vi "AutobalanceTest.vi"() -> ()   [LabVIEW 2009]
uses:
  Test Utilities/DAQ Read Actions.ctl
panel:
  in  "Log Name":string="Log"
  in  "Labels":string[](array[string])=["X1", "X2", "Y1", "Z1", "Z2", "Z3"]
  in  "Start":bool
  out "Servo Error vs Command Voltage":cluster{dbl[], dbl[]}[](graph)=[{[-9.0, 9.0, -8.8, 8.8, -8.6, 8.6, -8.4, 8.4, -8.2, 8.2, -8.0, 8.0, -7.8, 7.8, -7.6, 7.6, -7.4, 7.4, -7.2, 7.2, -7.0, 7.0, -6.8, 6.8, -6.6, 6.6, -6.4, 6.4, -6.199999999999999, 6.199999999999999, -6.0, 6.0, -5.8, 5.8, -5.6, 5.6, -5.4, 5.4, -5.199999999999999, 5.199999999999999, -5.0, 5.0, -4.8, 4.8, -4.6, 4.6, -4.3999999999999995, 4.3999999999999995, -4.199999999999999, 4.199999999999999, -4.0, 4.0, -3.8, 3.8, -3.5999999999999996, 3.5999999999999996, -3.3999999999999995, 3.3999999999999995, -3.1999999999999993, 3.1999999999999993, -3.0, 3.0, -2.8, 2.8, -2.5999999999999996, 2.5999999999999996, -2.3999999999999995, 2.3999999999999995, -2.1999999999999993, 2.1999999999999993, -2.0, 2.0, -1.7999999999999998, 1.7999999999999998, -1.5999999999999996, 1.5999999999999996, -1.3999999999999995, 1.3999999999999995, -1.1999999999999993, 1.1999999999999993, -1.0, 1.0, -0.7999999999999989, 0.7999999999999989, -0.5999999999999996, 0.5999999999999996, -0.40000000000000036, 0.40000000000000036, -0.1999999999999993, 0.1999999999999993, 0.0, -0.0, 0.20000000000000107, -0.20000000000000107, 0.40000000000000036, -0.40000000000000036, 0.6000000000000014, -0.6000000000000014, 0.8000000000000007, -0.8000000000000007], [5.23889540349607, -5.230763595763523, 5.259788534382426, -5.230763595763523, 5.259788534382426, -5.230763595763523, 5.259788534382426, -5.230763595763523, 5.259788534382426, -5.230763595763523, 5.259788534382426, -5.230763595763523, 5.259788534382426, -5.230763595763523, 5.259788534382426, -5.230763595763523, 5.259788534382426, -5.230763595763523, 5.259788534382426, -5.230763595763523, 5.259788534382426, -5.230763595763523, 5.259788534382426, -5.221320336306097, 5.259788534382426, -5.230763595763523, 5.259788534382426, -5.230763595763523, 5.259788534382426, -5.230763595763523, 5.259788534382426, -5.230763595763523, 5.259788534382426, -5.16630113951445, 5.259788534382426, -5.230763595763523, 5.259788534382426, -5.230763595763523, 5.259788534382426, -5.230763595763523, 5.259788534382426, -5.230763595763523, 5.259788534382426, -5.230763595763523, 5.259788534382426, -5.230763595763523, 5.259788534382426, -5.230763595763523, 5.259788534382426, -5.230763595763523, 5.259788534382426, -5.230763595763523, 5.259788534382426, -5.230763595763523, 5.259788534382426, -5.230763595763523, 5.259788534382426, -5.230763595763523, 5.259788534382426, -5.230763595763523, 5.259788534382426, -5.230763595763523, 5.259788534382426, -5.230763595763523, 5.259788534382426, -4.845854098653666, 5.259788534382426, -4.289184628066055, 5.259788534382426, -3.7257129745951536, 5.259788534382426, -3.1751435234854735, 5.259788534382426, -2.6188829711289623, 5.259788534382426, -2.060939148302728, 5.259788534382426, -1.502707977110508, 5.259788534382426, -0.9400082276367085, 5.187655957123444, -0.384859156987646, 4.632302266083261, 0.17346069172651984, 4.074197688727395, 0.731633238956068, 3.5206970694995556, 1.2900246998407006, 2.9635424103818933, 1.8498043247166114, 2.4063600794667632, 2.406408101449587, 1.8487558507937552, 2.963703818754653, 1.2906809935666468, 3.52138539517684, 0.732090775479772, 4.077071073464136, 0.1732899495896249, 4.629483544177946]}, {[-9.0, 9.0, -8.8, 8.8, -8.6, 8.6, -8.4, 8.4, -8.2, 8.2, -8.0, 8.0, -7.8, 7.8, -7.6, 7.6, -7.4, 7.4, -7.2, 7.2, -7.0, 7.0, -6.8, 6.8, -6.6, 6.6, -6.4, 6.4, -6.199999999999999, 6.199999999999999, -6.0, 6.0, -5.8, 5.8, -5.6, 5.6, -5.4, 5.4, -5.199999999999999, 5.199999999999999, -5.0, 5.0, -4.8, 4.8, -4.6, 4.6, -4.3999999999999995, 4.3999999999999995, -4.199999999999999, 4.199999999999999, -4.0, 4.0, -3.8, 3.8, -3.5999999999999996, 3.5999999999999996, -3.3999999999999995, 3.3999999999999995, -3.1999999999999993, 3.1999999999999993, -3.0, 3.0, -2.8, 2.8, -2.5999999999999996, 2.5999999999999996, -2.3999999999999995, 2.3999999999999995, -2.1999999999999993, 2.1999999999999993, -2.0, 2.0, -1.7999999999999998, 1.7999999999999998, -1.5999999999999996, 1.5999999999999996, -1.3999999999999995, 1.3999999999999995, -1.1999999999999993, 1.1999999999999993, -1.0, 1.0, -0.7999999999999989, 0.7999999999999989, -0.5999999999999996, 0.5999999999999996, -0.40000000000000036, 0.40000000000000036, -0.1999999999999993, 0.1999999999999993, 0.0, -0.0, 0.20000000000000107, -0.20000000000000107, 0.40000000000000036, -0.40000000000000036, 0.6000000000000014, -0.6000000000000014, 0.8000000000000007, -0.8000000000000007], [5.152580390546031, -5.227276646103857, 5.26040770497923, -5.227276646103857, 5.26040770497923, -5.227276646103857, 5.26040770497923, -5.227276646103857, 5.26040770497923, -5.227276646103857, 5.26040770497923, -5.227276646103857, 5.26040770497923, -5.227276646103857, 5.26040770497923, -5.227276646103857, 5.26040770497923, -5.227276646103857, 5.26040770497923, -5.227276646103857, 5.26040770497923, -5.227276646103857, 5.26040770497923, -5.227276646103857, 5.26040770497923, -5.227276646103857, 5.26040770497923, -5.227276646103857, 5.26040770497923, -5.227276646103857, 5.26040770497923, -5.227276646103857, 5.26040770497923, -5.227276646103857, 5.26040770497923, -5.227276646103857, 5.26040770497923, -5.227276646103857, 5.26040770497923, -5.227276646103857, 5.26040770497923, -5.227276646103857, 5.26040770497923, -5.227276646103857, 5.26040770497923, -5.227276646103857, 5.26040770497923, -5.227276646103857, 5.26040770497923, -5.227276646103857, 5.26040770497923, -5.227276646103857, 5.26040770497923, -5.227276646103857, 5.26040770497923, -5.227276646103857, 5.26040770497923, -5.227276646103857, 5.26040770497923, -5.227276646103857, 5.26040770497923, -5.227276646103857, 5.26040770497923, -5.227276646103857, 5.26040770497923, -5.227276646103857, 5.26040770497923, -5.227276646103857, 5.26040770497923, -5.227276646103857, 5.26040770497923, -5.227276646103857, 4.816100382863346, -5.227276646103857, 4.260788212659925, -4.689983459408686, 3.702119994547174, -4.130341645084159, 3.143975863465393, -3.5725983342860803, 2.5869591993094327, -3.0123466274812487, 2.0252975529047488, -2.4527984149741333, 1.4666902965914954, -1.8942823506166409, 0.9067132372667402, -1.3337585183451834, 0.346412507383714, -0.7734385785006557, -0.21321378403756536, -0.21338047871550267, -0.7731812018723434, 0.3462444789604288, -1.3341652540340105, 0.9074333608468415, -1.8933128500205254, 1.4660888578297582, -2.452686395199743, 2.0262683946413556]}, {[-9.0, 9.0, -8.8, 8.8, -8.6, 8.6, -8.4, 8.4, -8.2, 8.2, -8.0, 8.0, -7.8, 7.8, -7.6, 7.6, -7.4, 7.4, -7.2, 7.2, -7.0, 7.0, -6.8, 6.8, -6.6, 6.6, -6.4, 6.4, -6.199999999999999, 6.199999999999999, -6.0, 6.0, -5.8, 5.8, -5.6, 5.6, -5.4, 5.4, -5.199999999999999, 5.199999999999999, -5.0, 5.0, -4.8, 4.8, -4.6, 4.6, -4.3999999999999995, 4.3999999999999995, -4.199999999999999, 4.199999999999999, -4.0, 4.0, -3.8, 3.8, -3.5999999999999996, 3.5999999999999996, -3.3999999999999995, 3.3999999999999995, -3.1999999999999993, 3.1999999999999993, -3.0, 3.0, -2.8, 2.8, -2.5999999999999996, 2.5999999999999996, -2.3999999999999995, 2.3999999999999995, -2.1999999999999993, 2.1999999999999993, -2.0, 2.0, -1.7999999999999998, 1.7999999999999998, -1.5999999999999996, 1.5999999999999996, -1.3999999999999995, 1.3999999999999995, -1.1999999999999993, 1.1999999999999993, -1.0, 1.0, -0.7999999999999989, 0.7999999999999989, -0.5999999999999996, 0.5999999999999996, -0.40000000000000036, 0.40000000000000036, -0.1999999999999993, 0.1999999999999993, 0.0, -0.0, 0.20000000000000107, -0.20000000000000107, 0.40000000000000036, -0.40000000000000036, 0.6000000000000014, -0.6000000000000014, 0.8000000000000007, -0.8000000000000007], [4.959596256668532, -5.230473004384964, 5.259328112503975, -5.230473004384964, 5.259328112503975, -5.230473004384964, 5.259328112503975, -5.230473004384964, 5.185106744034811, -5.230473004384964, 5.259328112503975, -5.230473004384964, 5.259328112503975, -5.230473004384964, 5.259328112503975, -5.230473004384964, 5.259328112503975, -5.230473004384964, 5.159015256340536, -5.230473004384964, 5.259328112503975, -5.230473004384964, 5.259328112503975, -5.230473004384964, 5.259328112503975, -5.230473004384964, 5.259328112503975, -5.230473004384964, 5.129325305329152, -5.230473004384964, 5.259328112503975, -5.230473004384964, 5.259328112503975, -5.230473004384964, 5.259328112503975, -5.230473004384964, 5.259328112503975, -5.230473004384964, 5.259328112503975, -5.230473004384964, 5.259328112503975, -5.230473004384964, 5.259328112503975, -5.230473004384964, 5.255926632242481, -5.230473004384964, 5.259328112503975, -5.230473004384964, 5.259328112503975, -5.230473004384964, 5.2229389627275555, -5.230473004384964, 4.673812504480437, -5.230473004384964, 4.0734465222532945, -5.230473004384964, 3.555245852979843, -5.230473004384964, 3.0004917049265756, -5.230473004384964, 2.4339653771109324, -5.230473004384964, 1.878780464705355, -5.230473004384964, 1.2866940552275707, -5.230473004384964, 0.754889700982242, -5.230473004384964, 0.196855767024016, -5.230473004384964, -0.36771178764436996, -5.230473004384964, -0.9267665664635142, -5.230473004384964, -1.5072059928617625, -5.230473004384964, -2.04998339650814, -5.230473004384964, -2.6104255244754646, -5.230473004384964, -3.173707593912726, -5.230473004384964, -3.734434938746076, -5.230473004384964, -4.301727907705938, -5.230473004384964, -4.85368238083756, -5.230473004384964, -5.230473004384964, -5.230473004384964, -5.230473004384964, -5.230473004384964, -5.230473004384964, -5.230473004384964, -5.230473004384964, -4.853585007497255, -5.230473004384964, -4.2938007145633375, -5.230473004384964, -3.7419685785778927]}, {[-9.0, 9.0, -8.8, 8.8, -8.6, 8.6, -8.4, 8.4, -8.2, 8.2, -8.0, 8.0, -7.8, 7.8, -7.6, 7.6, -7.4, 7.4, -7.2, 7.2, -7.0, 7.0, -6.8, 6.8, -6.6, 6.6, -6.4, 6.4, -6.199999999999999, 6.199999999999999, -6.0, 6.0, -5.8, 5.8, -5.6, 5.6, -5.4, 5.4, -5.199999999999999, 5.199999999999999, -5.0, 5.0, -4.8, 4.8, -4.6, 4.6, -4.3999999999999995, 4.3999999999999995, -4.199999999999999, 4.199999999999999, -4.0, 4.0, -3.8, 3.8, -3.5999999999999996, 3.5999999999999996, -3.3999999999999995, 3.3999999999999995, -3.1999999999999993, 3.1999999999999993, -3.0, 3.0, -2.8, 2.8, -2.5999999999999996, 2.5999999999999996, -2.3999999999999995, 2.3999999999999995, -2.1999999999999993, 2.1999999999999993, -2.0, 2.0, -1.7999999999999998, 1.7999999999999998, -1.5999999999999996, 1.5999999999999996, -1.3999999999999995, 1.3999999999999995, -1.1999999999999993, 1.1999999999999993, -1.0, 1.0, -0.7999999999999989, 0.7999999999999989, -0.5999999999999996, 0.5999999999999996, -0.40000000000000036, 0.40000000000000036, -0.1999999999999993, 0.1999999999999993, 0.0, -0.0, 0.20000000000000107, -0.20000000000000107, 0.40000000000000036, -0.40000000000000036, 0.6000000000000014, -0.6000000000000014, 0.8000000000000007, -0.8000000000000007], [5.256829724339877, -5.233059557560193, 5.256829724339877, -5.233059557560193, 5.256829724339877, -5.233059557560193, 5.256829724339877, -5.233059557560193, 5.256829724339877, -5.233059557560193, 5.256829724339877, -5.233059557560193, 5.256829724339877, -5.233059557560193, 5.256829724339877, -5.233059557560193, 5.256829724339877, -5.233059557560193, 5.256829724339877, -5.233059557560193, 5.256829724339877, -5.233059557560193, 5.256829724339877, -5.187123226632507, 5.256829724339877, -5.233059557560193, 5.256829724339877, -5.233059557560193, 5.256829724339877, -5.233059557560193, 5.256829724339877, -5.233059557560193, 5.256829724339877, -5.101425908796338, 5.256829724339877, -5.233059557560193, 5.256829724339877, -5.233059557560193, 5.256829724339877, -5.233059557560193, 5.256829724339877, -5.233059557560193, 5.256829724339877, -5.233059557560193, 5.256829724339877, -5.233059557560193, 5.256829724339877, -4.936656824400534, 5.256829724339877, -4.370399092014139, 5.256829724339877, -3.8263928007871306, 5.256829724339877, -3.270996877809388, 5.256829724339877, -2.7166289891030306, 5.256829724339877, -2.156995323677104, 5.256829724339877, -1.5922699703924323, 5.256829724339877, -1.0415447894743053, 5.256829724339877, -0.48424056880896965, 5.256829724339877, 0.07133224979590863, 5.256829724339877, 0.632233057806092, 5.256829724339877, 1.195557503273296, 5.256829724339877, 1.7476477068567777, 5.256829724339877, 2.30553359483775, 5.256829724339877, 2.8609420009333033, 5.256829724339877, 3.419190420136921, 5.256829724339877, 3.9777585897998433, 5.256829724339877, 4.5316317524903456, 5.256829724339877, 5.086841120407304, 5.256829724339877, 5.256829724339877, 5.256829724339877, 5.256829724339877, 5.256829724339877, 5.256829724339877, 5.256829724339877, 5.256829724339877, 5.256829724339877, 5.256829724339877, 5.256829724339877, 5.256829724339877, 5.256829724339877, 5.256829724339877, 5.086719733562182, 5.256829724339877]}, {[-9.0, 9.0, -8.8, 8.8, -8.6, 8.6, -8.4, 8.4, -8.2, 8.2, -8.0, 8.0, -7.8, 7.8, -7.6, 7.6, -7.4, 7.4, -7.2, 7.2, -7.0, 7.0, -6.8, 6.8, -6.6, 6.6, -6.4, 6.4, -6.199999999999999, 6.199999999999999, -6.0, 6.0, -5.8, 5.8, -5.6, 5.6, -5.4, 5.4, -5.199999999999999, 5.199999999999999, -5.0, 5.0, -4.8, 4.8, -4.6, 4.6, -4.3999999999999995, 4.3999999999999995, -4.199999999999999, 4.199999999999999, -4.0, 4.0, -3.8, 3.8, -3.5999999999999996, 3.5999999999999996, -3.3999999999999995, 3.3999999999999995, -3.1999999999999993, 3.1999999999999993, -3.0, 3.0, -2.8, 2.8, -2.5999999999999996, 2.5999999999999996, -2.3999999999999995, 2.3999999999999995, -2.1999999999999993, 2.1999999999999993, -2.0, 2.0, -1.7999999999999998, 1.7999999999999998, -1.5999999999999996, 1.5999999999999996, -1.3999999999999995, 1.3999999999999995, -1.1999999999999993, 1.1999999999999993, -1.0, 1.0, -0.7999999999999989, 0.7999999999999989, -0.5999999999999996, 0.5999999999999996, -0.40000000000000036, 0.40000000000000036, -0.1999999999999993, 0.1999999999999993, 0.0, -0.0, 0.20000000000000107, -0.20000000000000107, 0.40000000000000036, -0.40000000000000036, 0.6000000000000014, -0.6000000000000014, 0.8000000000000007, -0.8000000000000007], [5.263974822618488, -5.227400981912923, 5.263974822618488, -5.227400981912923, 5.263974822618488, -5.227400981912923, 5.263974822618488, -5.227400981912923, 5.263974822618488, -5.227400981912923, 5.263974822618488, -5.227400981912923, 5.263974822618488, -5.227400981912923, 5.263974822618488, -5.227400981912923, 5.263974822618488, -5.227400981912923, 5.263974822618488, -5.227400981912923, 5.263974822618488, -5.227400981912923, 5.263974822618488, -5.227400981912923, 5.263974822618488, -5.227400981912923, 5.263974822618488, -5.227400981912923, 5.263974822618488, -5.227400981912923, 5.263974822618488, -5.227400981912923, 5.263974822618488, -5.148952658429211, 5.263974822618488, -5.227400981912923, 5.263974822618488, -5.227400981912923, 5.263974822618488, -5.227400981912923, 5.263974822618488, -5.227400981912923, 5.263974822618488, -5.227400981912923, 5.263974822618488, -5.227400981912923, 5.263974822618488, -5.227400981912923, 5.263974822618488, -5.220561113431062, 5.263974822618488, -4.921752419879671, 5.263974822618488, -4.3688845907808185, 5.263974822618488, -3.807650554575446, 5.263974822618488, -3.2511568020263124, 5.263974822618488, -2.685828673761237, 5.263974822618488, -2.1314919673965056, 5.263974822618488, -1.5748082227549012, 5.263974822618488, -1.01374101680912, 5.263974822618488, -0.45373380599704494, 5.263974822618488, 0.11014870611018425, 5.263974822618488, 0.6669815591105563, 5.263974822618488, 1.225626084602838, 5.263974822618488, 1.786107034122924, 5.263974822618488, 2.344951298222356, 5.263974822618488, 2.9050771545212695, 5.263974822618488, 3.4637371750479877, 5.263974822618488, 4.022005979258876, 5.263974822618488, 4.5798562601446395, 5.263974822618488, 5.135883901198011, 5.263974822618488, 5.263974822618488, 5.263974822618488, 5.263974822618488, 5.263974822618488, 5.263974822618488, 5.1360866861896906, 5.263974822618488, 4.57979088949585, 5.263974822618488, 4.022218098114356, 5.263974822618488]}, {[-9.0, 9.0, -8.8, 8.8, -8.6, 8.6, -8.4, 8.4, -8.2, 8.2, -8.0, 8.0, -7.8, 7.8, -7.6, 7.6, -7.4, 7.4, -7.2, 7.2, -7.0, 7.0, -6.8, 6.8, -6.6, 6.6, -6.4, 6.4, -6.199999999999999, 6.199999999999999, -6.0, 6.0, -5.8, 5.8, -5.6, 5.6, -5.4, 5.4, -5.199999999999999, 5.199999999999999, -5.0, 5.0, -4.8, 4.8, -4.6, 4.6, -4.3999999999999995, 4.3999999999999995, -4.199999999999999, 4.199999999999999, -4.0, 4.0, -3.8, 3.8, -3.5999999999999996, 3.5999999999999996, -3.3999999999999995, 3.3999999999999995, -3.1999999999999993, 3.1999999999999993, -3.0, 3.0, -2.8, 2.8, -2.5999999999999996, 2.5999999999999996, -2.3999999999999995, 2.3999999999999995, -2.1999999999999993, 2.1999999999999993, -2.0, 2.0, -1.7999999999999998, 1.7999999999999998, -1.5999999999999996, 1.5999999999999996, -1.3999999999999995, 1.3999999999999995, -1.1999999999999993, 1.1999999999999993, -1.0, 1.0, -0.7999999999999989, 0.7999999999999989, -0.5999999999999996, 0.5999999999999996, -0.40000000000000036, 0.40000000000000036, -0.1999999999999993, 0.1999999999999993, 0.0, -0.0, 0.20000000000000107, -0.20000000000000107, 0.40000000000000036, -0.40000000000000036, 0.6000000000000014, -0.6000000000000014, 0.8000000000000007, -0.8000000000000007], [5.263480094674747, -5.226487348935504, 5.263480094674747, -5.226487348935504, 5.263480094674747, -5.226487348935504, 5.263480094674747, -5.226487348935504, 5.263480094674747, -5.226487348935504, 5.263480094674747, -5.226487348935504, 5.263480094674747, -5.226487348935504, 5.263480094674747, -5.226487348935504, 5.263480094674747, -5.226487348935504, 5.263480094674747, -5.226487348935504, 5.263480094674747, -5.226487348935504, 5.263480094674747, -5.226487348935504, 5.263480094674747, -5.226487348935504, 5.263480094674747, -5.226487348935504, 5.263480094674747, -5.226487348935504, 5.263480094674747, -5.226487348935504, 5.263480094674747, -5.1686018069424255, 5.263480094674747, -5.226487348935504, 5.263480094674747, -5.226487348935504, 5.263480094674747, -5.226487348935504, 5.263480094674747, -5.226487348935504, 5.263480094674747, -5.226487348935504, 5.263480094674747, -5.226487348935504, 5.263480094674747, -5.226487348935504, 5.263480094674747, -5.193187596490152, 5.263480094674747, -4.637811518038858, 5.263480094674747, -4.081206984502, 5.263480094674747, -3.524034917017728, 5.263480094674747, -2.9627505301425683, 5.263480094674747, -2.4027526353192177, 5.263480094674747, -1.8424705396576762, 5.263480094674747, -1.2828518864055751, 5.263480094674747, -0.7242520828425978, 5.263480094674747, -0.16136168949490276, 5.263480094674747, 0.3988479992764996, 5.263480094674747, 0.9594242206317586, 5.263480094674747, 1.5204810838359601, 5.263480094674747, 2.0793902776149884, 5.263480094674747, 2.640436891620216, 5.263480094674747, 3.199210545132962, 5.263480094674747, 3.7596575689539073, 5.263480094674747, 4.317666294701486, 5.263480094674747, 4.875694454765391, 5.263480094674747, 5.263480094674747, 5.263480094674747, 5.263480094674747, 5.263480094674747, 5.263480094674747, 5.263480094674747, 5.263480094674747, 5.263480094674747, 5.263480094674747, 4.8763560814319336, 5.263480094674747, 4.318407948335608, 5.263480094674747]}]
  in  "Max Volts":dbl=9.0
  out "Text Output File":path=path "C:/Documents and Settings/mbletzin/Desktop/Work/OM Source/CraneBayOneBox_30_300.000_100_10.txt"
  out "Result Sample":dbl[](array[numeric])=[-0.8000000000000007, 4.629483544177946, 2.0262683946413556, -3.7419685785778927, 5.256829724339877, 5.263974822618488, 5.263480094674747]
  in  "milliseconds to wait":u32=10
  in  "Command Voltage Task":refnum<k21>="Command Voltage"
  in  "samples per channel":i32=30
  in  "rate":dbl=300.0 caption="Samples per Second" format="%0.2f"
  in  "Servo Error Task":refnum<k21>="Servo Errors"
  in  "Number of Increments":i32=100
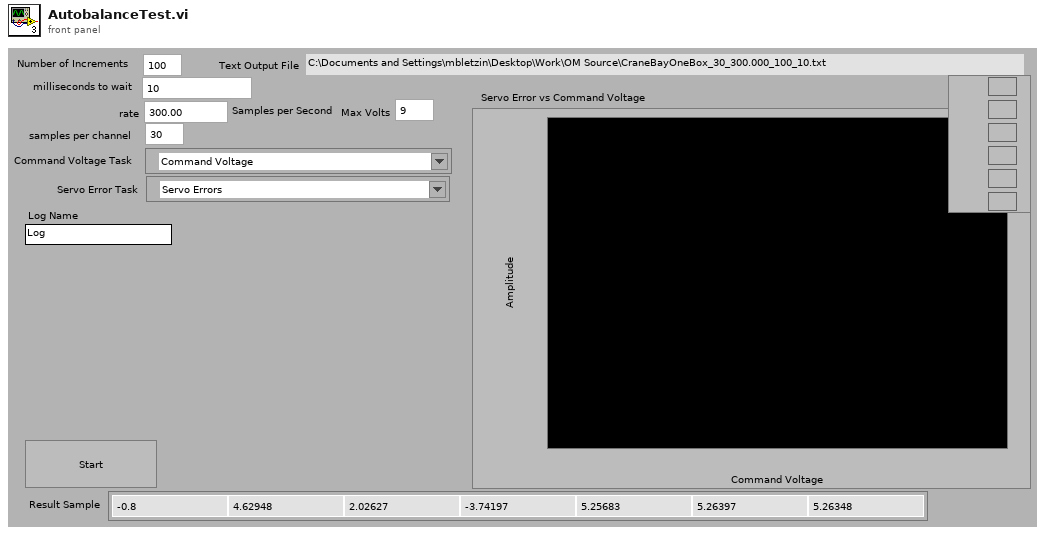
[diagram p1: front panel]
types:
  T1 = typedef "DAQ Read Actions.ctl" = enum16{"Start", "Read", "Stop"}
  T2 = enum16{"open", "replace", "create", "open or create", "replace or create", "replace or create with confirmation"}
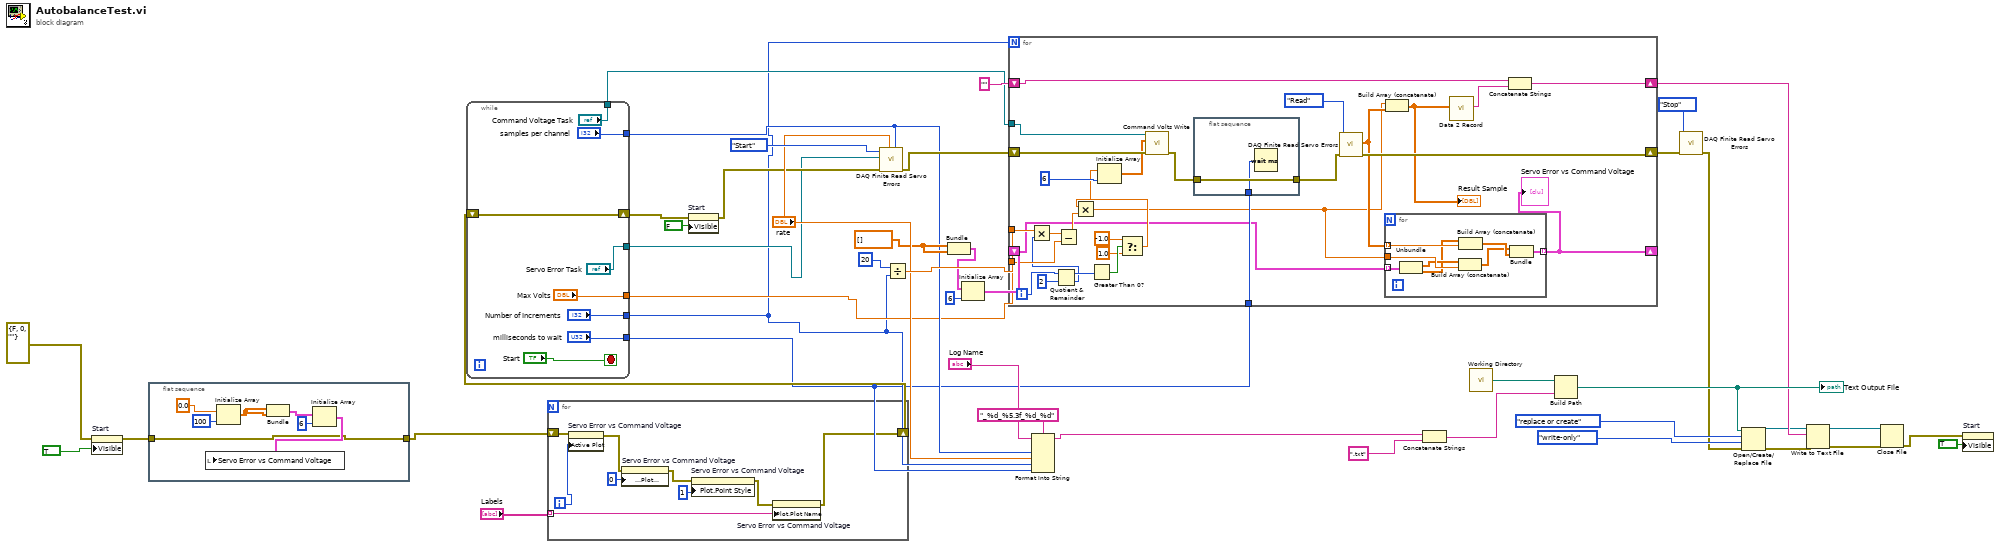
[diagram p0: block diagram]
diagram:
  w20 = dbl[] []
  n1 = property on="Start" class="Bool"(error in=errorcluster {"status"=FALSE, "code"=0, "source"=""} ("error out"), "Visible"=TRUE) -> (error out=w2:errorcluster)  [unwired: 1 in, 1 out]
  n2 = flat-sequence {
    tunnel: w2 -> [w45]
    tunnel: [w45] -> w1
    frame #0 {
      n3 = Initialize Array(0.0, 100 ("dimension size")) -> (w49:dbl[])
      n4 = Bundle(w49, w49) -> (w47:cluster{dbl[], dbl[]})  [unwired: 1 in]
      n5 = Initialize Array(w47, 6 ("dimension size")) -> (w46:cluster{dbl[], dbl[]}[])
      n6 = local write "Servo Error vs Command Voltage"(w46) -> ()
    }
  }
  n7 = for {
    shift-right: [w53] -> w14
    shift-left: w1 -> [w55]
    tunnel: "Labels" -> [w52] mode=indexing
    i -> [w60]
    n8 = property on="Servo Error vs Command Voltage" class="XYGraph (strict)"(error in=w55, "Active Plot"=w60) -> (error out=w58:errorcluster)  [unwired: 1 in, 1 out]
    n9 = property on="Servo Error vs Command Voltage" class="XYGraph (strict)"(error in=w58, "Plot.Plot Interpolation"=u8 0) -> (error out=w57:errorcluster)  [unwired: 1 in, 1 out]
    n10 = property on="Servo Error vs Command Voltage" class="XYGraph (strict)"(error in=w57, "Plot.Point Style"=u8 1) -> (error out=w54:errorcluster)  [unwired: 1 in, 1 out]
    n11 = property on="Servo Error vs Command Voltage" class="XYGraph (strict)"(error in=w54, "Plot.Plot Name"=w52) -> (error out=w53:errorcluster)  [unwired: 1 in, 1 out]
  }
  n12 = while {
    tunnel: ["Servo Error Task"] -> w8
    tunnel: ["Command Voltage Task"] -> w7
    tunnel: ["samples per channel"] -> w6
    tunnel: ["Max Volts"] -> w5
    tunnel: ["Number of Increments"] -> w4
    tunnel: ["milliseconds to wait"] -> w3
    shift-right: [w61] -> w17
    shift-left: w14 -> [w61]
    stop <- "Start" stop-if-true
  }
  n13 = property on="Start" class="Bool"(error in=w17, "Visible"=FALSE) -> (error out=w15:errorcluster)  [unwired: 1 in, 1 out]
  n14 = call "DAQ Finite Read Servo Errors.vi"("samples per channel"=w6, "rate"="rate", "error in"=w15, "task/channels in"=w8, "Action"=DAQ_Read_Actions."Start") -> ("error out"=w41:errorcluster)  [unwired: 6 out]
  n15 = Divide(x=20, y=w4) -> (x/y=w42:dbl)
  n16 = Bundle(w20, w20) -> (w19:cluster{dbl[], dbl[]})  [unwired: 1 in]
  n17 = Initialize Array(w19, 6 ("dimension size")) -> (w18:cluster{dbl[], dbl[]}[])
  n18 = for {
    N: w4 -> [_]
    tunnel: w42 -> [w97]
    tunnel: w7 -> [w93]
    shift-right: [w90] -> w25
    shift-left: w41 -> [w92]
    tunnel: w3 -> [w83]
    shift-right: [w84] -> w30
    shift-left: "" -> [w82]
    tunnel: w5 -> [w95]
    shift-right: [w70] -> _
    shift-left: w18 -> [w69]
    i -> [w81]
    n19 = Quotient & Remainder(x=w81, y=2) -> (x-y*floor(x/y)=w79:i32, floor(x/y)=w74:i32)
    n20 = Multiply(x=w97, y=w74) -> (x*y=w96:dbl)
    n21 = Subtract(x=w96, y=w95) -> (x-y=w73:dbl)
    n22 = Greater Than 0?(x=w79) -> (x > 0?=w78:bool)
    n23 = Select(t=-1.0, s=w78, f=1.0) -> (s? t:f=w75:dbl)
    n24 = Multiply(x=w75, y=w73) -> (x*y=w71:dbl)
    n25 = Initialize Array(w71, 6 ("dimension size")) -> (w87:dbl[])
    n26 = call "Command Volts Write.vi"("error in"=w92, "Command Volts"=w87, "task/channels in"=w93) -> ("error out"=w89:errorcluster)  [unwired: 8 out]
    n27 = flat-sequence {
      tunnel: w89 -> [w107]
      tunnel: [w107] -> w88
      tunnel: w83 -> [w106]
      frame #0 {
        n28 = Wait (ms)(milliseconds to wait=w106) -> ()  [unwired: 1 out]
      }
    }
    n29 = call "DAQ Finite Read Servo Errors.vi"("error in"=w88, "Action"=DAQ_Read_Actions."Read") -> ("error out"=w90:errorcluster, "Average"=w72:dbl[])  [unwired: 3 in, 5 out]
    n30 = for {
      tunnel: w72 -> [w104] mode=indexing
      tunnel: w71 -> [w105]
      tunnel: [w101] -> w70 mode=indexing
      tunnel: w69 -> [w100] mode=indexing
      n31 = Unbundle(w100) -> (w99:dbl[], w98:dbl[])
      n32 = Build Array (concatenate)(w99, w105) -> (w102:dbl[])
      n33 = Build Array (concatenate)(w98, w104) -> (w103:dbl[])
      n34 = Bundle(w102, w103) -> (w101:cluster{dbl[], dbl[]})  [unwired: 1 in]
    }
    "Servo Error vs Command Voltage" <- w70
    n35 = Build Array (concatenate)(w71, w72) -> (w86:dbl[])
    "Result Sample" <- w86
    n36 = call "Data 2 Record.vi"("Data"=w86) -> ("Records"=w85:string)  [unwired: 2 in, 8 out]
    n37 = Concatenate Strings(w82, w85) -> (w84:string)
  }
  n38 = Format Into String(format string="_%d_%5.3f_%d_%d", initial string="Log Name", w6, "rate", w4, w3) -> (resulting string=w38:string)  [unwired: 1 in, 1 out]
  n39 = Concatenate Strings(w38, ".txt" ("string")) -> (w33:string)
  n40 = call "Working Directory.vi"() -> ("Path"=w34:path)  [unwired: 1 out]
  n41 = Build Path(base path=w34, name or relative path=w33) -> (appended path=w35:path)
  "Text Output File" <- w35
  n42 = call "DAQ Finite Read Servo Errors.vi"("error in"=w25, "Action"=DAQ_Read_Actions."Stop") -> ("error out"=w24:errorcluster)  [unwired: 3 in, 6 out]
  n43 = Open/Create/Replace File(file path (use dialog)=w35, error in=w24, operation (0:open)=T2."replace or create", access (0:read/write)=enum16{"read/write", "read-only", "write-only"}."write-only") -> (refnum out=w29:refnum<file>, error out=w28:errorcluster)  [unwired: 3 out]
  n44 = Write to Text File(file (use dialog)=w29, text=w30, error in=w28) -> (refnum out=w27:refnum<file>, error out=w26:errorcluster)  [unwired: 2 out]
  n45 = Close File(refnum=w27, error in=w26) -> (error out=w12:errorcluster)  [unwired: 1 out]
  n46 = property on="Start" class="Bool"(error in=w12, "Visible"=TRUE) -> ()  [unwired: 1 in, 2 out]
